vi "Actor Core.vi"(8 "error in":errorcluster, 11 "Normal Entry Console View In":refnum<class "Normal Entry Console View.lvclass">) -> (0 "error out":errorcluster, 3 "Actor out":refnum<class "Actor.lvclass">)   [LabVIEW 2019, in "Normal Entry Console View.lvclass"]
doc: "(<B>Filename</B>: Actor Framework.lvlib:Actor.lvclass:Actor Core.vi)\n\nReceives messages to the actor, reacts to them, and initiates any error handling that may shut the actor down.\n\nDescendant classes may override this VI to append parallel tasks for the actor to complete while it handles messages. Overrides use the Call Parent Method node.\n\n<License>\nCopyright © 2017 Composed Systems, LLC | All rights reserved\nwww.composed.io\n\nAuthor: Ethan Stern <ethan.stern@composed.io>\n\nThis software is provided \"AS IS\" WITHOUT WARRANTIES, either express or implied, AND IS FOR EDUCATIONAL PURPOSES ONLY.\n</License>"
uses:
  <vilib>/gpm_packages/@cs/Car-wash/Source/Normal Entry Console View/Normal Entry Console View/Normal Entry Console View.lvclass
  C:/Program Files/National Instruments/LabVIEW 2019/vi.lib/gpm_packages/@cs/Car-wash/Source/Entry Console View Definition/Entry Console View Definition/Entry Console View Definition.lvclass
  <vilib>/ActorFramework/Actor/Actor.lvclass
  <vilib>/gpm_packages/@cs/Car-wash/Source/Entry Console View Definition/Entry Console View Definition/Entry Console View Definition.lvclass
panel:
  in  "High Pressure Wash":bool
  in  "Spot Free Rinse":bool
  in  "Low Pressure Wax":bool
  in  "Bug Remover":bool
  in  "Pre-Soak":bool
  in  "Tire Shine Foam":bool
  in  "Air Dry":bool
  in  "Under Body Wash":bool
  in  "Start":bool
  # "Entry Console"
  # "Wash Options"
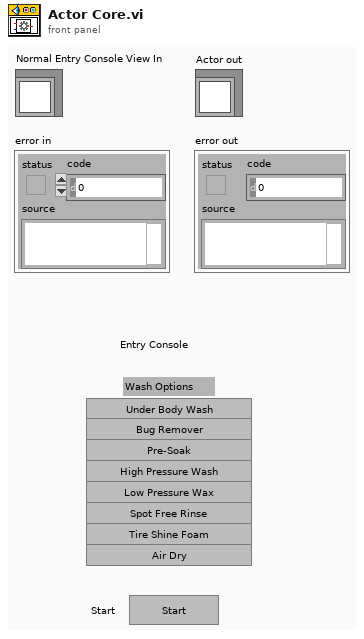
[diagram p1: front panel]
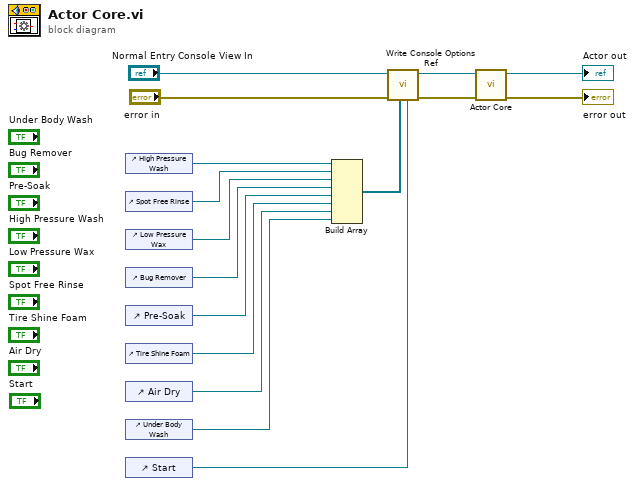
[diagram p0: block diagram]
diagram:
  n1 = control-ref of="High Pressure Wash"() -> (w10:refnum<vi>)
  n2 = control-ref of="Spot Free Rinse"() -> (w8:refnum<vi>)
  n3 = control-ref of="Low Pressure Wax"() -> (w7:refnum<vi>)
  n4 = control-ref of="Bug Remover"() -> (w6:refnum<vi>)
  n5 = control-ref of="Pre-Soak"() -> (w5:refnum<vi>)
  n6 = control-ref of="Tire Shine Foam"() -> (w4:refnum<vi>)
  n7 = control-ref of="Air Dry"() -> (w3:refnum<vi>)
  n8 = control-ref of="Under Body Wash"() -> (w2:refnum<vi>)
  n9 = control-ref of="Start"() -> (w1:refnum<vi>)
  n10 = Build Array(w10, w8, w7, w6, w5, w4, w3, w2) -> (w9:refnum<vi>[])
  n11 = call <vilib>:"Write Console Options Ref.vi"("Start Ref"=w1, "Console Options"=w9, "Entry Console View Definition in"="Normal Entry Console View In") -> ("Entry Console View Definition out"=w11:refnum<class "Normal Entry Console View.lvclass">)  [unwired: 8 in]
  n12 = call-parent "Actor Core.vi"("error in"="error in", "Entry Console View Definition In"=w11) -> ("error out"=→"error out":errorcluster, "Actor out"=→"Actor out":refnum<class "Actor.lvclass">)  [unwired: 8 in]
